vi "OccupancyEstimators.vi"() -> ()   [LabVIEW 2011]
uses:
  Dependencies/global.vi
panel:
  out "fAirInletValve":dbl
  out "Estimated Occupancy":u32
  out "fRoomTemperature":dbl
  out "fRoomCO2":dbl
  out "fAirInletCO2":dbl
  out "fAirInletTemperature":dbl
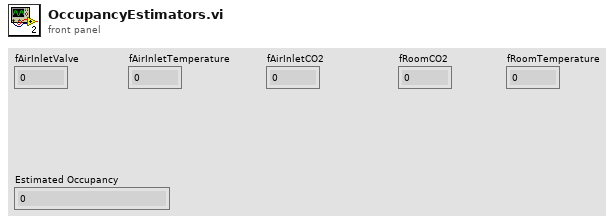
[diagram p1: front panel]
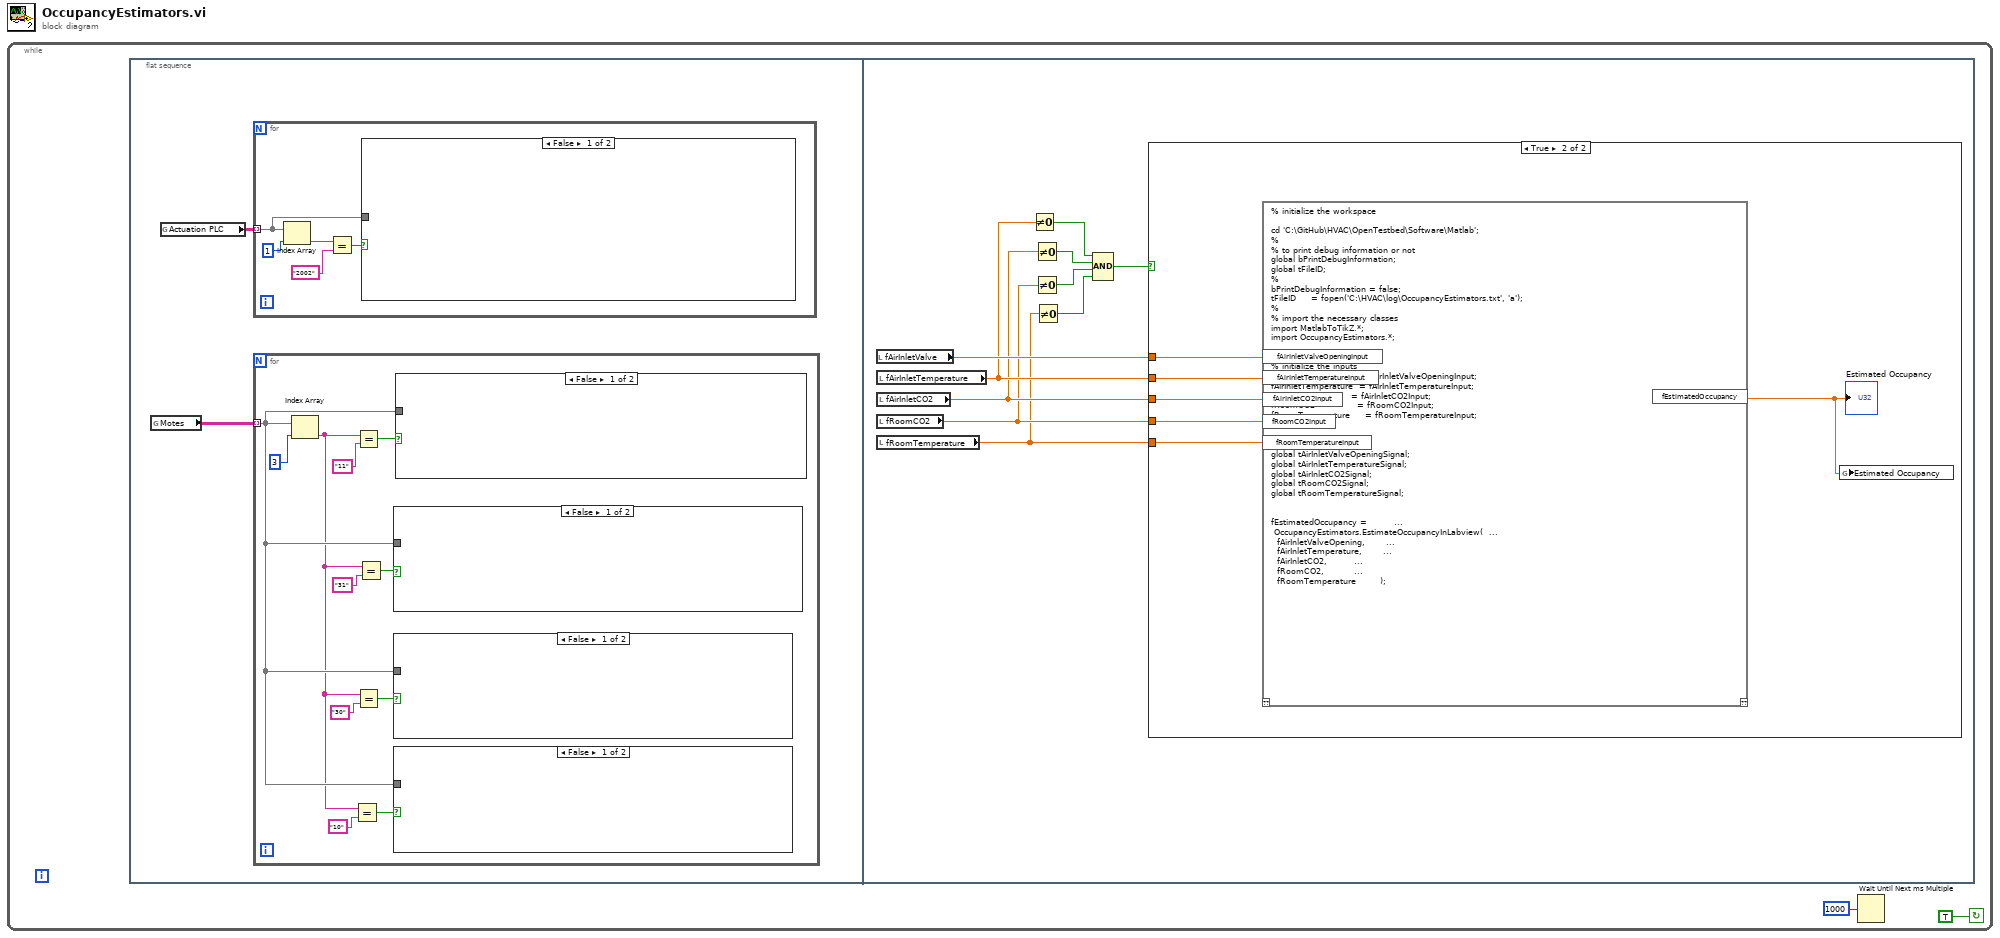
[diagram p0: block diagram]
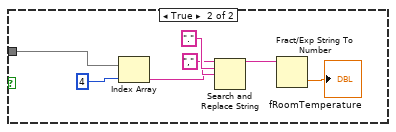
[diagram p2: hidden frame]
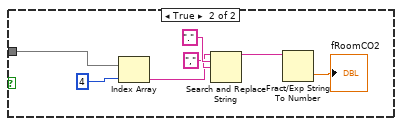
[diagram p3: hidden frame]
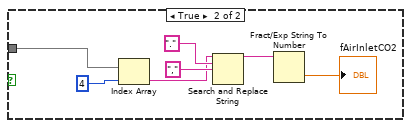
[diagram p4: hidden frame]
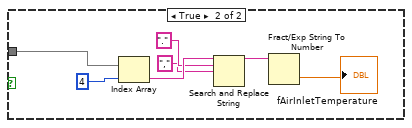
[diagram p5: hidden frame]
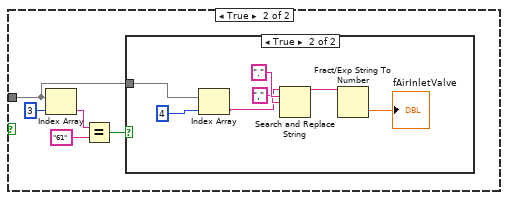
[diagram p6: hidden frame]
diagram:
  n1 = while {
    stop <- TRUE continue-if-true
    n2 = flat-sequence {
      frame #0 {
        n3 = global read "global.vi" "Motes"() -> (w3:string[][])
        n4 = global read "global.vi" "Actuation PLC"() -> (w4:string[][])
        n5 = for {
          tunnel: w4 -> [w44] mode=indexing
          n6 = Index Array(array=w44, index=1) -> (element=w47:string)
          n7 = Equal?(x=w47, y="2002") -> (x = y?=w45:bool)
          n8 = case shown="False" w45 {
            tunnel: w44 -> [_ w49]
            frame False {
            }
            frame True {
              n9 = Index Array(array=w49, index=3) -> (element=w52:string)
              n10 = Equal?(x=w52, y="61") -> (x = y?=w50:bool)
              n11 = case shown="True" w50 {
                tunnel: w49 -> [_ w60]
                frame False {
                }
                frame True {
                  n12 = Index Array(array=w60, index=4) -> (element=w54:string)
                  n13 = Search and Replace String(input string=w54, search string=".", replace string="," ("replace string (\"\")")) -> (result string=w55:string)  [unwired: 5 in, 3 out]
                  n14 = Fract/Exp String To Number(string=w55) -> (number=→"fAirInletValve":dbl)  [unwired: 3 in, 1 out]
                }
              }
            }
          }
        }
        n15 = for {
          tunnel: w3 -> [w8] mode=indexing
          n16 = Index Array(array=w8, index=3) -> (element=w5:string)
          n17 = Equal?(x=w5, y="10") -> (x = y?=w6:bool)
          n18 = Equal?(x=w5, y="11") -> (x = y?=w13:bool)
          n19 = Equal?(x=w5, y="30") -> (x = y?=w9:bool)
          n20 = Equal?(x=w5, y="31") -> (x = y?=w12:bool)
          n21 = case shown="False" w12 {
            tunnel: w8 -> [_ w34]
            frame False {
            }
            frame True {
              n22 = Index Array(array=w34, index=4) -> (element=w30:string)
              n23 = Search and Replace String(input string=w30, search string=".", replace string="," ("replace string (\"\")")) -> (result string=w31:string)  [unwired: 5 in, 3 out]
              n24 = Fract/Exp String To Number(string=w31) -> (number=→"fAirInletCO2":dbl)  [unwired: 3 in, 1 out]
            }
          }
          n25 = case shown="False" w9 {
            tunnel: w8 -> [_ w27]
            frame False {
            }
            frame True {
              n26 = Index Array(array=w27, index=4) -> (element=w23:string)
              n27 = Search and Replace String(input string=w23, search string=".", replace string="," ("replace string (\"\")")) -> (result string=w24:string)  [unwired: 5 in, 3 out]
              n28 = Fract/Exp String To Number(string=w24) -> (number=→"fRoomCO2":dbl)  [unwired: 3 in, 1 out]
            }
          }
          n29 = case shown="False" w6 {
            tunnel: w8 -> [_ w20]
            frame False {
            }
            frame True {
              n30 = Index Array(array=w20, index=4) -> (element=w16:string)
              n31 = Search and Replace String(input string=w16, search string=".", replace string="," ("replace string (\"\")")) -> (result string=w17:string)  [unwired: 5 in, 3 out]
              n32 = Fract/Exp String To Number(string=w17) -> (number=→"fRoomTemperature":dbl)  [unwired: 3 in, 1 out]
            }
          }
          n33 = case shown="False" w13 {
            tunnel: w8 -> [_ w42]
            frame False {
            }
            frame True {
              n34 = Index Array(array=w42, index=4) -> (element=w41:string)
              n35 = Search and Replace String(input string=w41, search string=".", replace string="," ("replace string (\"\")")) -> (result string=w38:string)  [unwired: 5 in, 3 out]
              n36 = Fract/Exp String To Number(string=w38) -> (number=→"fAirInletTemperature":dbl)  [unwired: 3 in, 1 out]
            }
          }
        }
      }
      frame #1 {
        n37 = local read "fAirInletValve"() -> (w70:dbl)
        n38 = local read "fAirInletTemperature"() -> (w69:dbl)
        n39 = local read "fAirInletCO2"() -> (w68:dbl)
        n40 = local read "fRoomCO2"() -> (w67:dbl)
        n41 = local read "fRoomTemperature"() -> (w66:dbl)
        n42 = Not Equal To 0?(x=w69) -> (x != 0?=w65:bool)
        n43 = Not Equal To 0?(x=w68) -> (x != 0?=w64:bool)
        n44 = Not Equal To 0?(x=w67) -> (x != 0?=w63:bool)
        n45 = Not Equal To 0?(x=w66) -> (x != 0?=w62:bool)
        n46 = Compound Arithmetic op=AND(w65, w64, w63, w62) -> (w61:bool)
        n47 = case shown="True" w61 {
          tunnel: w70 -> [_ w75]
          tunnel: w69 -> [_ w74]
          tunnel: w68 -> [_ w73]
          tunnel: w67 -> [_ w72]
          tunnel: w66 -> [_ w71]
          frame False {
          }
          frame True {
            n48 = script code="% initialize the workspace\n\ncd 'C:\\GitHub\\HVAC\\OpenTestbed\\Software\\Matlab';\n%\n% to print debug information or not\nglobal bPrintDebugInformation;\nglobal tFileID;\n%\nbPrintDebugInformation\t= false;\ntFileID\t\t\t\t\t= fopen('C:\\HVAC\\log\\OccupancyEstimators.txt', 'a');\n%\n% import the necessary classes\nimport MatlabToTikZ.*;\nimport OccupancyEstimators.*;\n\n\n% initialize the inputs\nfAirInletValveOpening = fAirInletValveOpeningInput;\nfAirInletTemperature  = fAirInletTemperatureInput;\nfAirInletCO2           = fAirInletCO2Input;\nfRoomCO2              = fRoomCO2Input;\nfRoomTemperature     = fRoomTemperatureInput;\n\n\nglobal tEstimator;\nglobal tAirInletValveOpeningSignal;\nglobal tAirInletTemperatureSignal;\nglobal tAirInletCO2Signal;\nglobal tRoomCO2Signal;\nglobal tRoomTemperatureSignal;\n\n\nfEstimatedOccupancy =\t\t\t\t\t\t\t\t\t...\n\tOccupancyEstimators.EstimateOccupancyInLabview(\t\t...\n\t\tfAirInletValveOpening,\t\t\t\t\t\t\t...\n\t\tfAirInletTemperature,\t\t\t\t\t\t\t...\n\t\tfAirInletCO2,\t\t\t\t\t\t\t\t\t...\n\t\tfRoomCO2,\t\t\t\t\t\t\t\t\t\t...\n\t\tfRoomTemperature\t\t\t\t\t\t\t\t);"("fAirInletValveOpeningInput"=w75, "fAirInletTemperatureInput"=w74, "fAirInletCO2Input"=w73, "fRoomCO2Input"=w72, "fRoomTemperatureInput"=w71) -> ("fEstimatedOccupancy"=w76:dbl)  [unwired: 1 in, 1 out]
            "Estimated Occupancy" <- w76
            n49 = global write "global.vi" "Estimated Occupancy"(w76) -> ()
          }
        }
      }
    }
    n50 = Wait Until Next ms Multiple(millisecond multiple=u32 1000) -> ()  [unwired: 1 out]
  }
